vi "Save uS GUI as JPG.vi"(8 "error in (no error)":errorcluster, 10 "Path to JPG file":path, 11 "Father of all uServices in":refnum<class "Father of all uServices.lvclass">) -> (0 "error out":errorcluster, 3 "Father of all uServices out":refnum<class "Father of all uServices.lvclass">)   [LabVIEW 2026, in "TALOS.lvlib" / "Father of all uServices.lvlib" / "Father of all uServices.lvclass"]
uses:
  Father of all uServices.lvclass
  C:/LabVIEW Code/TALOS/talos/Ancestor/Ancestor/Ancestor.lvclass
  Ancestor/Ancestor/Ancestor.lvclass/Ancestor.ctl
  Classes/uService List/uService List.lvclass/uService List.ctl
  Ancestor/Ancestor/Read ID.vi
  Support VIs/Generate Error.vi
  FGV/Error Memory/Get Error Description.vi
  Support VIs/Get PC name.vi
  Support VIs/Get Class Name.vi
  <vilib>/Utility/error.llb/Clear Errors.vi
  FGV/Error Memory/Error Memory Core.vi
  <vilib>/AdvancedString/Delimited String to 1D String Array.vi
  <vilib>/AdvancedString/Delimited String to 1D String Array (string).vi
  Support VIs/Circus Root Path.vi
  FGV/Error Memory/Error Crt Lvl checker.vi
  FGV/Error Memory/Error Memory Core.vi/40c8088d-b597-4017-91af-faa98e00292e.vi
  FGV/Error Memory/Error Memory Core.vi/d4a3ab98-063c-4e44-b43d-fbdcfe6c2be2.vi
  Support VIs/Global Memory.vi
  <vilib>/Utility/LVClass/Get LV Class Name.vi
  Support VIs/Is in Packed Library.vi
  Support VIs/TALOS Root path.vi
  Support VIs/Read CSV worksheet.vi
  Support VIs/Global Constants.vi
  <vilib>/Utility/error.llb/General Error Handler.vi
  Support VIs/Error Log.vi
  Classes/uService List/uService List.lvclass
  Ancestor/Ancestor/Ancestor.lvclass
  <vilib>/Comparison/Equal/Equal Functor/Equal Functor.lvclass
  TALOS.lvlib
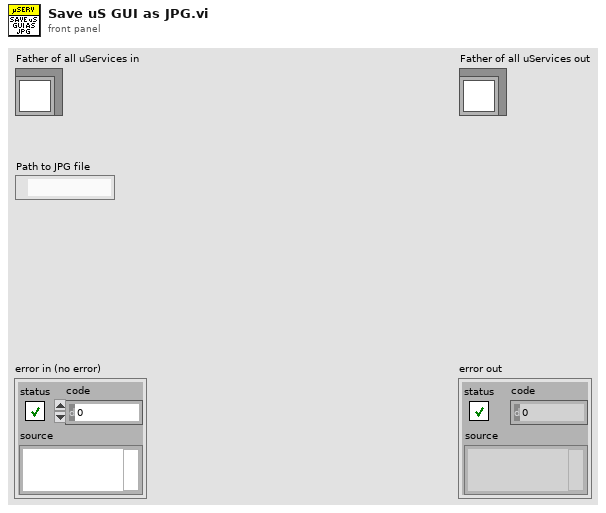
[diagram p1: front panel]
types:
  T1 = typedef "imagedata.ctl" = cluster{"image type":i32, "image depth":i32, "image":u8[], "mask":u8[], "colors":u32[], "Rectangle":cluster{"left":i16, "top":i16, "right":i16, "bottom":i16}}
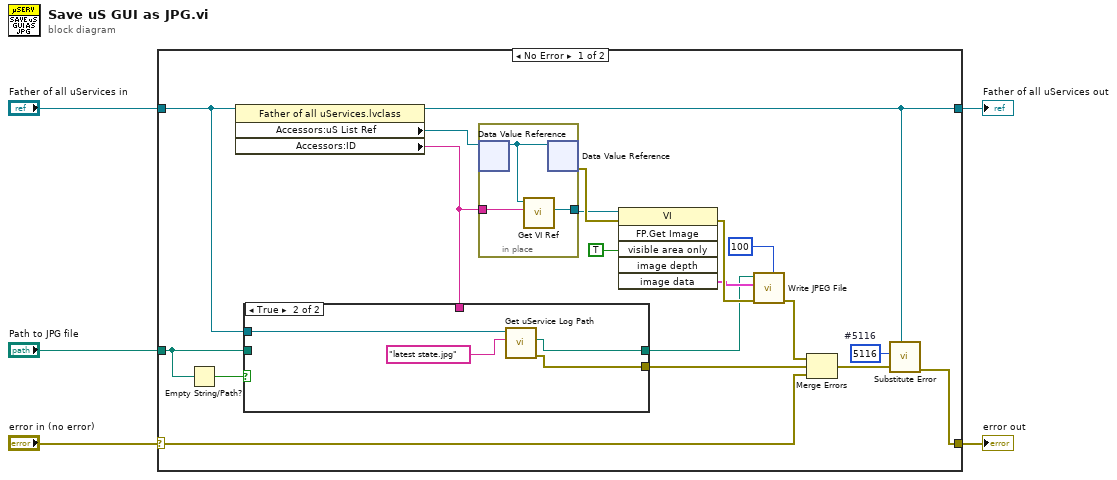
[diagram p0: block diagram]
diagram:
  n1 = case shown="No Error" "error in (no error)" {
    selector: "error in (no error)" -> [w13 w34]
    tunnel: [w9 w34] -> w4
    tunnel: [w8 w33] -> w2
    tunnel: "Father of all uServices in" -> [w6 w33]
    tunnel: "Path to JPG file" -> [w11 _]
    frame No Error {
      w7 = 5116  # #5116
      n2 = Empty String/Path?(string/path=w11) -> (empty?=w12:bool)
      n3 = property class="Father of all uServices.lvclass"(reference=w6) -> (reference out=w8:refnum<class "Father of all uServices.lvclass">, "Accessors:uS List Ref"=w21:refnum<data-value>, "Accessors:ID"=w20:string)  [unwired: 1 in, 1 out]
      n4 = case shown="True" w12 {
        tunnel: [_ w26] -> w24
        tunnel: w20 -> [_ _]
        tunnel: [w25 w27] -> w15
        tunnel: w11 -> [w25 _]
        tunnel: w6 -> [_ w29]
        frame False {
        }
        frame True {
          n5 = call "Get uService Log Path.vi"("Log File Suffix"="latest state.jpg", "Father of all uServices in"=w29) -> ("error out"=w26:errorcluster, "Log File Path"=w27:path)  [unwired: 7 in, 1 out]
        }
      }
      n6 = in-place {
        in-place-border: w20 -> [w31]
        in-place-border: [w30] -> w18
        n7 = in-place-dvr #1(w21) -> (w32:refnum<class "uService List.lvclass">)  [unwired: 1 out]
        n8 = call "Get VI Ref.vi"("ID"=w31, "uService List in"=w32) -> ("Vi Ref"=w30:refnum<vi>)  [unwired: 7 in, 2 out]
        n9 = in-place-dvr #1(w32) -> (w22:errorcluster)  [unwired: 1 out]
      }
      n10 = invoke class="VI" method="FP.Get Image"(reference=w18, error in=w22, "visible area only"=TRUE ("Visible Area Only")) -> (error out=w23:errorcluster, "image data"=w16:T1)  [unwired: 3 in, 4 out]
      n11 = call <vilib>:"Write JPEG File.vi"("quality (80)"=100, "error in (no error)"=w23, "image data"=w16, "path to JPEG file"=w15) -> ("error out"=w14:errorcluster)  [unwired: 6 in, 1 out]
      n12 = Merge Errors(w14, w24, w13) -> (w10:errorcluster)
      n13 = call "Substitute Error.vi"("LabVIEW Object"=w8, "error in (no error)"=w10, "Error Code"=w7) -> ("error out"=w9:errorcluster)  [unwired: 8 in]
    }
    frame Error {
    }
  }
  "error out" <- w4
  "Father of all uServices out" <- w2
